vi "PSAE_VCH_Path.vi"() -> (2 "All Path":cluster{"Tree PNG":path, "Data":path})   [LabVIEW 2016]
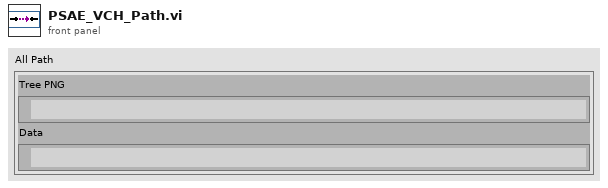
[diagram p1: front panel]
types:
  T1 = enum32{"invalid app kind", "Development System", "Run Time System", "Student Edition", "Embedded LabVIEW", "Evaluation", "Custom"}
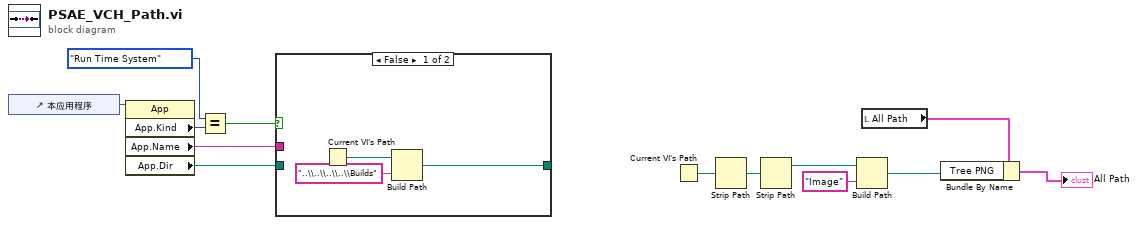
[diagram p0: block diagram]
diagram:
  n1 = control-ref of="本应用程序"() -> (w13:refnum<vi>)
  n2 = property class="App"(reference=w13) -> ("App.Kind"=w12:T1, "App.Name"=w9:string, "App.Dir"=w8:path)  [unwired: 1 in, 2 out]
  n3 = Equal?(x=T1."Run Time System" ("应用程序:类别"), y=w12) -> (x = y?=w10:bool)
  n4 = case shown="False" w10 {
    tunnel: w9 -> [_ _]
    tunnel: w8 -> [_ w17]
    tunnel: [w15 w17] -> _
    frame False {
      n5 = Current VI's Path() -> (path=w16:path)
      n6 = Build Path(base path=w16, name or relative path="..\\..\\..\\..\\Builds") -> (appended path=w15:path)
    }
    frame True {
    }
  }
  n7 = Current VI's Path() -> (path=w3:path)
  n8 = Strip Path(path=w3) -> (stripped path=w2:path)  [unwired: 1 out]
  n9 = Strip Path(path=w2) -> (stripped path=w1:path)  [unwired: 1 out]
  n10 = Build Path(base path=w1, name or relative path="Image") -> (appended path=w5:path)
  n11 = local read "All Path"() -> (w6:cluster{"Tree PNG":path, "Data":path})
  n12 = Bundle By Name(cluster=w6, "Tree PNG"=w5) -> (→"All Path":cluster{"Tree PNG":path, "Data":path})
